vi "Set tds Factor.vi"(8 "error in (no error)":errorcluster, 9 "tds Factor":dbl, 10 "Channel":T1, 11 "EPU452 in":refnum<class "EPU452.lvclass">) -> (0 "error out":errorcluster, 2 "Response":string, 3 "EPU452 out":refnum<class "EPU452.lvclass">)   [LabVIEW 2018, in "EPU452.lvclass"]
uses:
  EPU452.lvclass
  Controls/Channels.ctl
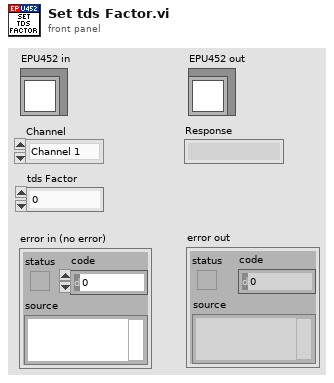
[diagram p1: front panel]
types:
  T1 = typedef "EPU452.lvclass/Channels.ctl" = enum16{"Channel 1", "Channel 2", "Channel 3", "Channel 4"}
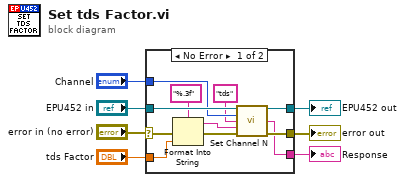
[diagram p0: block diagram]
diagram:
  n1 = case shown="No Error" "error in (no error)" {
    selector: "error in (no error)" -> [w13 w20]
    tunnel: [w16 w20] -> w6
    tunnel: [w17 w19] -> w4
    tunnel: "EPU452 in" -> [w18 w19]
    tunnel: "Channel" -> [w15 _]
    tunnel: "tds Factor" -> [w10 _]
    tunnel: [w8 _] -> w1
    frame No Error {
      n2 = Format Into String(format string="%.3f", error in=w13, w10) -> (resulting string=w11:string, error out=w12:errorcluster)  [unwired: 1 in]
      n3 = call "Set Channel N.vi"("EPU452 in"=w18, "Channel"=w15, "Function"="tds", "Argument/s"=w11, "error in (no error)"=w12) -> ("EPU452 out"=w17:refnum<class "EPU452.lvclass">, "Response"=w8:string, "error out"=w16:errorcluster)  [unwired: 8 in]
    }
    frame Error {
    }
  }
  "error out" <- w6
  "EPU452 out" <- w4
  "Response" <- w1
